vi "Display Cetroids (SubVI).vi"(11 "Measurement data":T2={"CentroidX"=[335.1659288406372], "CentroidY"=[364.63495540618896], "I"=[], "Acquired Buffer Number"=9830}) -> (1 "Intensities":T1(graph)={"CentroidY[0]"=364.63495540618896, "CentroidY[1]"=0.0, "CentroidY[2]"=0.0, "CentroidY[3]"=0.0, "CentroidY[4]"=0.0, "CentroidY[5]"=0.0, "CentroidY[6]"=0.0, "CentroidY[7]"=0.0, "CentroidY[8]"=0.0}, 2 "Y pos":T1(graph)={"CentroidY[0]"=364.63495540618896, "CentroidY[1]"=0.0, "CentroidY[2]"=0.0, "CentroidY[3]"=0.0, "CentroidY[4]"=0.0, "CentroidY[5]"=0.0, "CentroidY[6]"=0.0, "CentroidY[7]"=0.0, "CentroidY[8]"=0.0}, 3 "X pos":T3(graph))   [LabVIEW 2011]
panel:
  out "size(s)":i32
  in  "Y scale factor":dbl=100.0
  in  "X scale factor \n(nm/pixel)":dbl=100.0
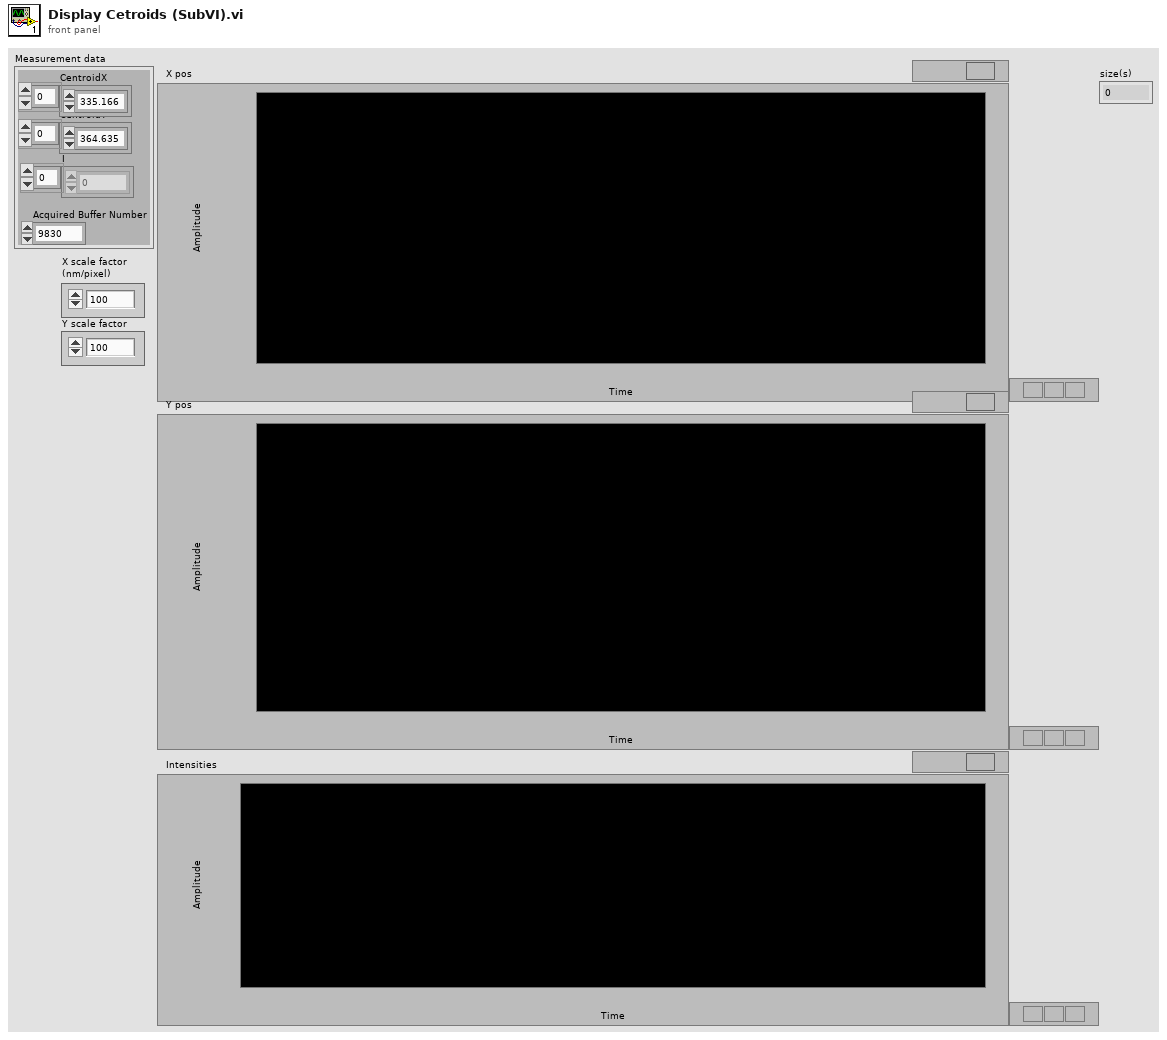
[diagram p1: front panel]
types:
  T1 = cluster{"CentroidY[0]":dbl, "CentroidY[1]":dbl, "CentroidY[2]":dbl, "CentroidY[3]":dbl, "CentroidY[4]":dbl, "CentroidY[5]":dbl, "CentroidY[6]":dbl, "CentroidY[7]":dbl, "CentroidY[8]":dbl}
  T2 = cluster{"CentroidX":dbl[], "CentroidY":dbl[], "I":dbl[], "Acquired Buffer Number":u32}
  T3 = cluster{"[0]":dbl, "[1]":dbl, "[2]":dbl, "[3]":dbl, "[4]":dbl, "[5]":dbl, "[6]":dbl, "[7]":dbl, "[8]":dbl}
  T4 = cluster{"I[0]":dbl, "I[1]":dbl, "I[2]":dbl, "I[3]":dbl, "I[4]":dbl, "I[5]":dbl, "I[6]":dbl, "I[7]":dbl, "I[8]":dbl}
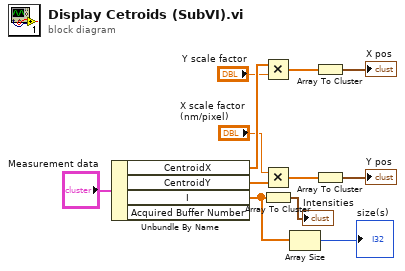
[diagram p0: block diagram]
diagram:
  n1 = Unbundle By Name("Measurement data") -> ("CentroidX"=w11:dbl[], "CentroidY"=w10:dbl[], "I"=w2:dbl[])  [unwired: 1 out]
  n2 = Multiply(x=w11, y="Y scale factor") -> (x*y=w9:dbl[])
  n3 = Multiply(x="X scale factor \n(nm/pixel)", y=w10) -> (x*y=w7:dbl[])
  n4 = Array To Cluster(array=w2) -> (cluster=→"Intensities":T4)
  n5 = Array Size(array=w2) -> (size(s)=→"size(s)":i32)
  n6 = Array To Cluster(array=w9) -> (cluster=→"X pos":T3)
  n7 = Array To Cluster(array=w7) -> (cluster=→"Y pos":T3)
